vi "READ_CAPACITOR.vi"(0 "Arduino Resource in":T3, 5 "Resitor":u32=4700, 7 "Resistor Pin":u8=13, 9 "Analog input Pin":u8, 11 "error in":errorcluster) -> (4 "Arduino Resource out":T3, 6 "Capacitor":dbl, 15 "error out":errorcluster)   [LabVIEW 2015]
uses:
  <vilib>/LabVIEW Interface for Arduino/Type Defs/Board Type.ctl
  <vilib>/LabVIEW Interface for Arduino/Type Defs/Connection Type.ctl
  <vilib>/LabVIEW Interface for Arduino/LabVIEW Interface for Arduino.lvlib
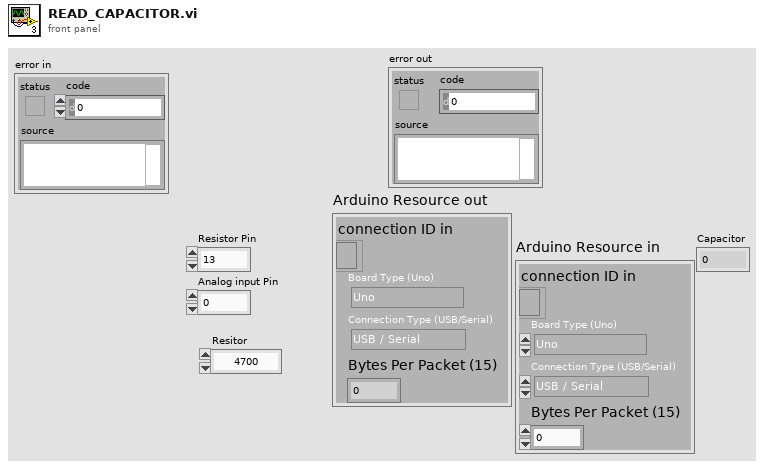
[diagram p1: front panel]
types:
  T1 = typedef "LabVIEW Interface for Arduino.lvlib/Board Type.ctl" = enum16{"Uno", "Dimuelanove w/Atmega 328", "Mega 2560"}
  T2 = typedef "LabVIEW Interface for Arduino.lvlib/Connection Type.ctl" = enum8{"USB / Serial", "XBEE", "BlueSmirf (Bluetooth)"}
  T3 = cluster{"connection ID in":refnum<k31>, "Board Type (Uno)":T1, "Connection Type (USB/Serial)":T2, "Bytes Per Packet (15)":u32}
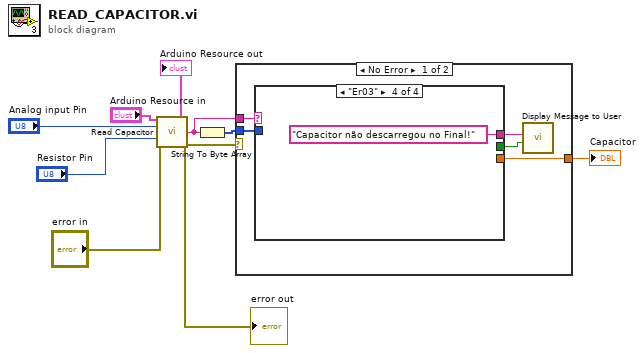
[diagram p0: block diagram]
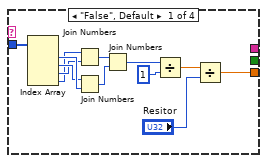
[diagram p2: hidden frame]
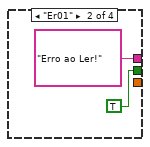
[diagram p3: hidden frame]
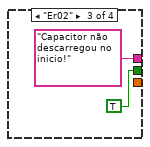
[diagram p4: hidden frame]
diagram:
  n1 = call "Read Capacitor.vi"("Arduino Resource in"="Arduino Resource in", "Analog input Pin"="Analog input Pin", "Resistor Pin"="Resistor Pin", "error in"="error in") -> ("Arduino Resource out"=→"Arduino Resource out":T3, "Time (us)"=w5:string, "error out"=w7:errorcluster)  [unwired: 9 in]
  "error out" <- w7
  n2 = String To Byte Array(string=w5) -> (unsigned byte array=w6:u8[])
  n3 = case shown="No Error" w7 {
    tunnel: w6 -> [w11 _]
    tunnel: w5 -> [w12 _]
    tunnel: [w10 _] -> w4
    frame No Error {
      n4 = case shown="\"Er03\"" w12 {
        tunnel: [_ "Erro ao Ler!" "Capacitor não descarregou no inicio!" "Capacitor não descarregou no Final!"] -> w14
        tunnel: [_ TRUE ("SAIR") TRUE ("SAIR") _] -> w13
        tunnel: w11 -> [w17 _ _ _]
        tunnel: [w16 _ _ _] -> w10
        frame "False", Default {
          n5 = Index Array(array=w17) -> (element #1=w23:u8, element #2=w22:u8, element #3=w21:u8, element #4=w20:u8)  [unwired: 4 in]
          n6 = Join Numbers(hi=w20, lo=w21) -> ((hi.lo)=w18:u16)
          n7 = Join Numbers(hi=w22, lo=w23) -> ((hi.lo)=w19:u16)
          n8 = Join Numbers(hi=w18, lo=w19) -> ((hi.lo)=w24:u32)
          n9 = Divide(x=w24, y=u32 1) -> (x/y=w26:dbl)
          n10 = Divide(x=w26, y="Resitor") -> (x/y=w16:dbl)
        }
        frame "Er01" {
        }
        frame "Er02" {
        }
        frame "Er03" {
        }
      }
      n11 = call "Display Message to User"("Enable"=w13, "Message"=w14) -> ()  [unwired: 8 in, 2 out]
    }
    frame Error {
    }
  }
  "Capacitor" <- w4
